vi "Current TimeRec.vi"() -> (0 "Current TimeRec":T1)   [LabVIEW 2009]
uses:
  TimeRec.ctl
panel:
  out "current time":timestamp
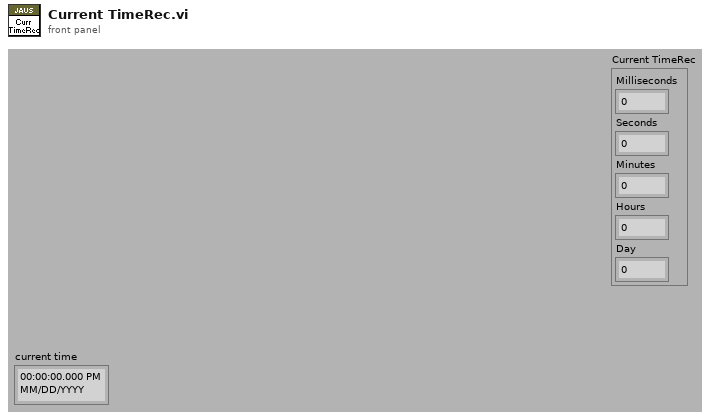
[diagram p1: front panel]
types:
  T1 = typedef "TimeRec.ctl" = cluster{"Milliseconds":u32, "Seconds":u32, "Minutes":u32, "Hours":u32, "Day":u32}
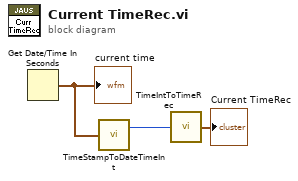
[diagram p0: block diagram]
diagram:
  n1 = Get Date/Time In Seconds() -> (seconds since 1Jan1904=w3:timestamp)
  "current time" <- w3
  n2 = call "TimeStampToDateTimeInt.vi"("Time Stamp"=w3) -> ("timeInt"=w2:u32)  [unwired: 1 out]
  n3 = call "TimeIntToTimeRec.vi"("Time Int"=w2) -> ("TimeRec"=→"Current TimeRec":T1)
